vi "Outgoing Messages.vi"(8 "error in (no error)":errorcluster, 11 "Node Ptr":T3 format="%.0x") -> (0 "error out":errorcluster)   [LabVIEW 2009, in "NI-XNET Custom Device.lvlib"]
uses:
  NI-XNET Custom Device.lvlib
  <vilib>/NI VeriStand/Custom Device API/Custom Device Item Ref.ctl
  Add Selected.ctl
  Add All.ctl
  <vilib>/xnet/xnet.llb/XNET String To IO Name (Cluster).vi
  <vilib>/NI VeriStand/Custom Device API/Get Item Property (String).vi
  <vilib>/NI VeriStand/Custom Device API/Set Item Property (Variant).vi
  <vilib>/NI VeriStand/Custom Device API/Custom Device API.lvlib
  Program Files/National Instruments/LabVIEW 2009/resource/objmgr/xnet.rc
panel:
  out "Channel Assignment":u32(ring)=1 items=["A"=1, "B"=2, "A and B"=3]
  out "Cycle Repetition":u32
  out "Channel Assignments":u32[](array[numeric])
  out "Identifiers":u32[](array[numeric])
  out "In Cycle Repetitions?":bool
  out "Preamble":bool
  out "Startup":bool
  out "Sync":bool
  in  "Header 4":cluster{"Section Name 2":string}={"Section Name 2"="FlexRay Specific Settings"}
  in  "Frame Selection":i32(listbox)
  in  "Add All":T1
  in  "Header 3":cluster{"Section Name 2":string}={"Section Name 2"="Frame Timing"}
  in  "Header 2":cluster{"Section Name 2":string}={"Section Name 2"="Frame Settings"}
  out "Default Payload":u8[](array[numeric])
  out "Transmit Time":dbl
  out "Timing Type":u32(ring) items=["Cyclic Data", "Event Data", "Cyclic Remote", "Event Remote"]
  out "Extended Identifier?":bool
  out "Payload Length":u32
  out "Identifier":u32
  in  "Add Frame":T2
  in  "Header":cluster{"Section Name":string}={"Section Name"="Frame Selection"}
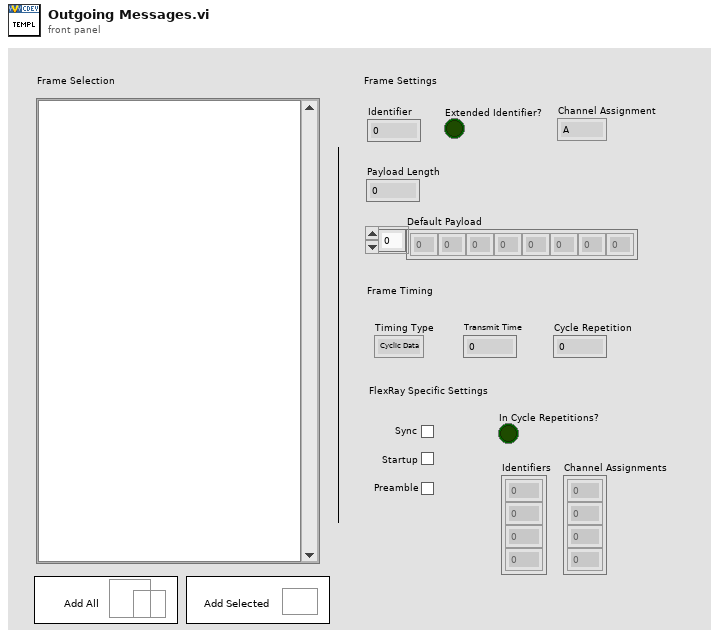
[diagram p1: front panel]
types:
  T1 = typedef "NI-XNET Custom Device.lvlib/Add All.ctl" = bool
  T2 = typedef "NI-XNET Custom Device.lvlib/Add Selected.ctl" = bool
  T3 = typedef "Custom Device API.lvlib/Custom Device Item Ref.ctl" = u64
  T4 = typedef "Custom Device API.lvlib/Custom Device Commands.ctl" = enum16{"Default", "Item renamed", "Shutdown"}
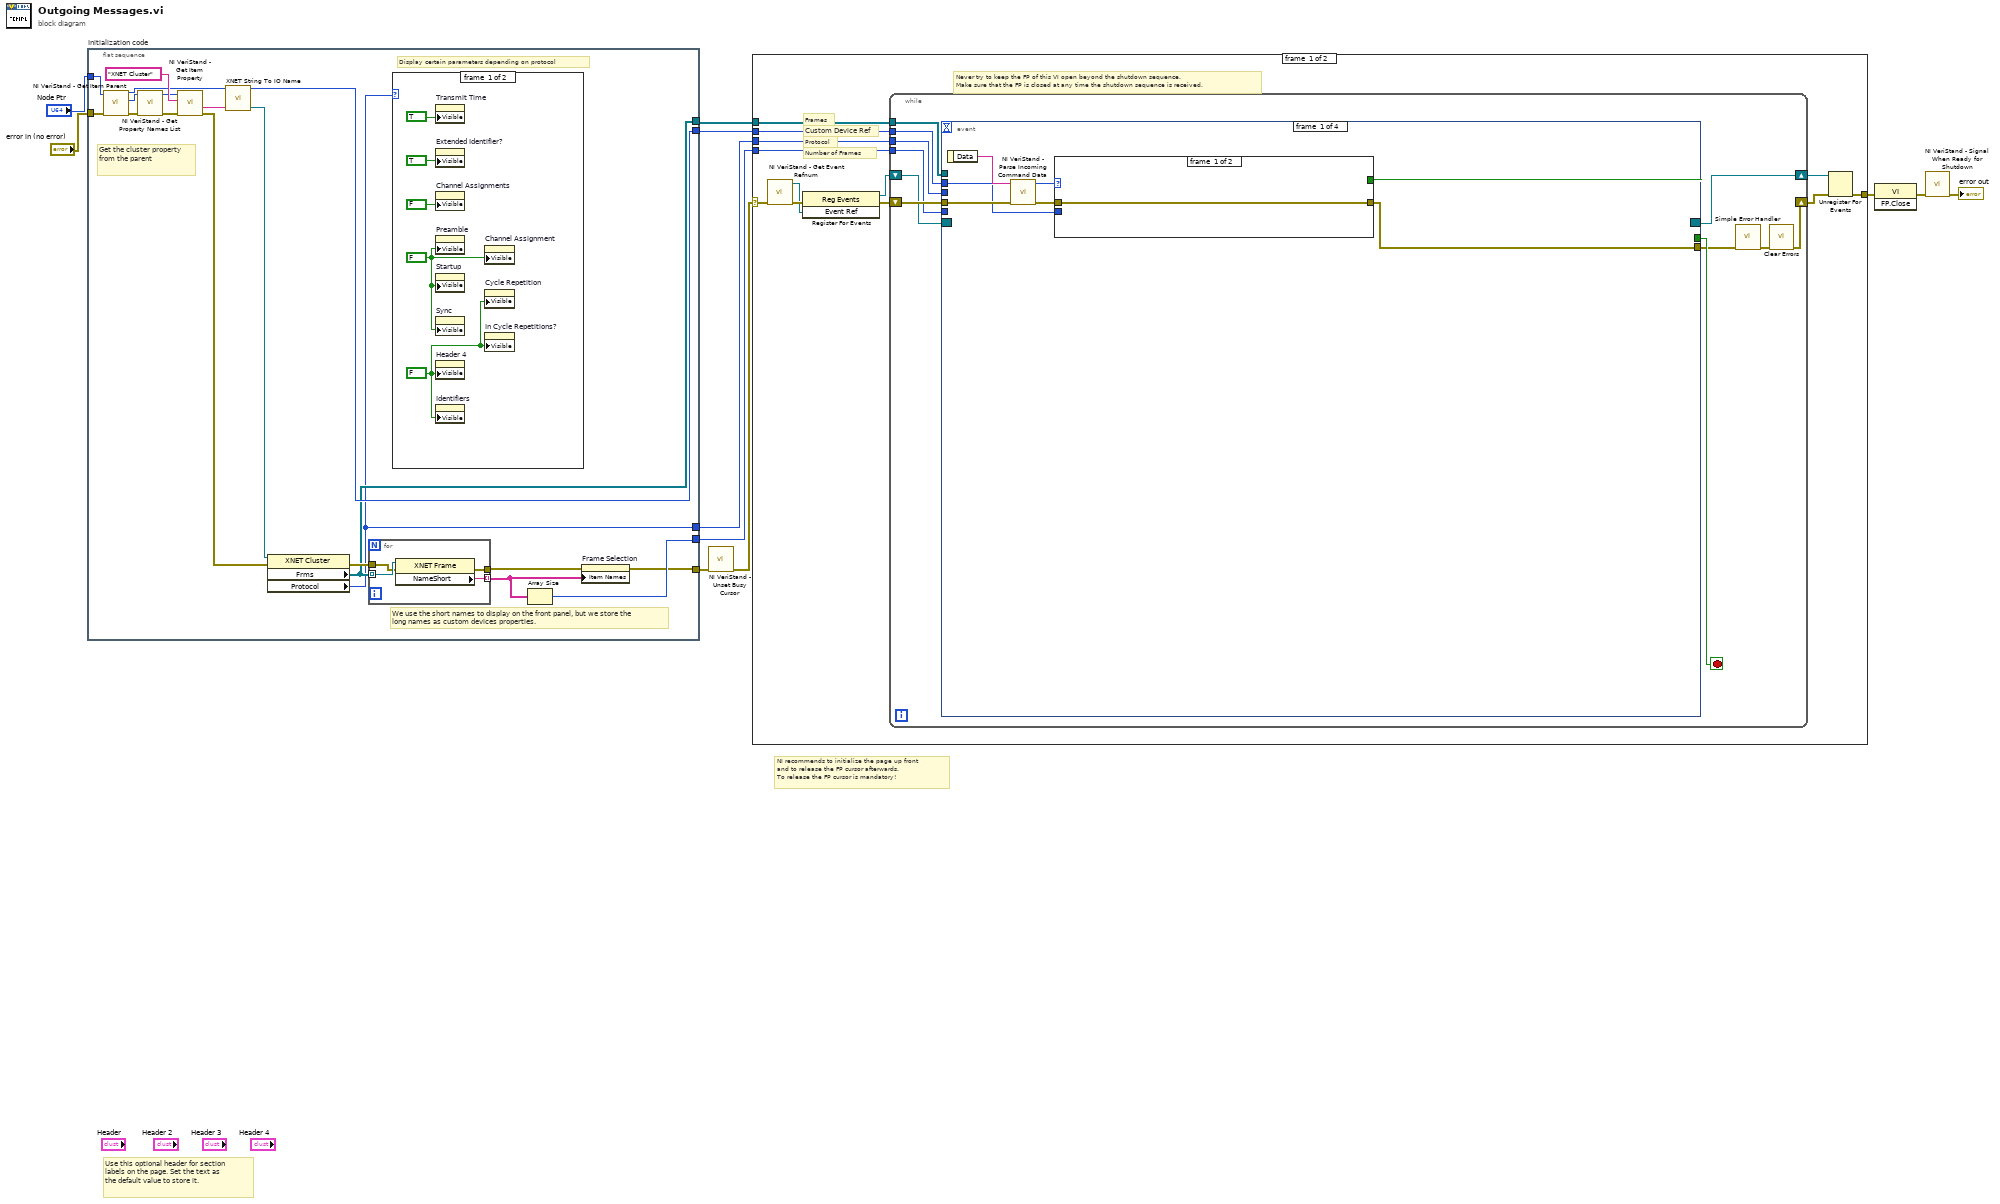
[diagram p0: block diagram]
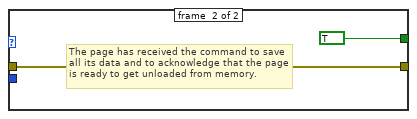
[diagram p2: hidden frame]
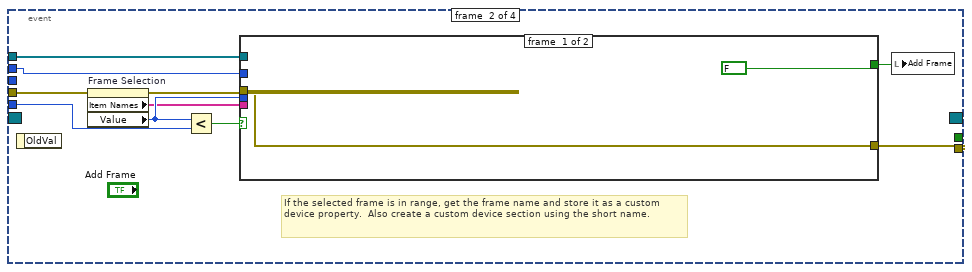
[diagram p3: hidden frame]
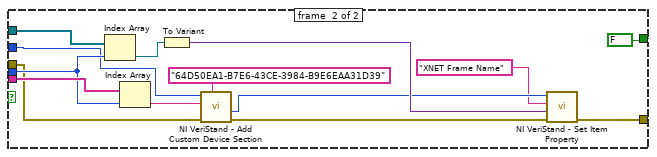
[diagram p4: hidden frame]
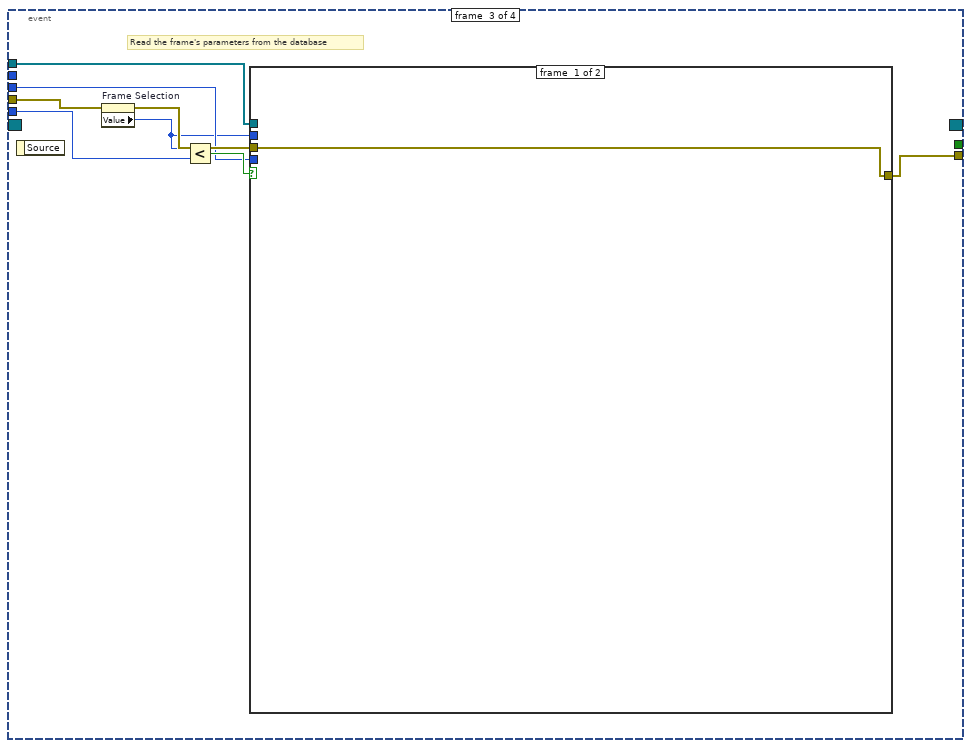
[diagram p5: hidden frame]
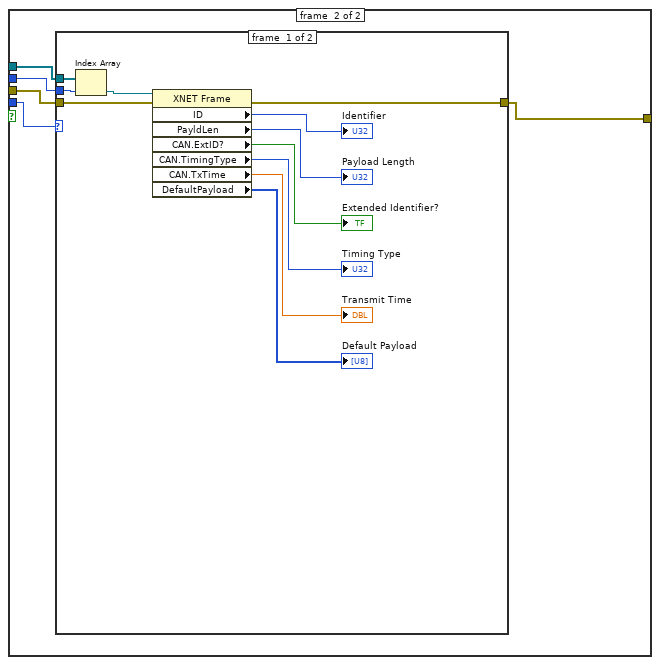
[diagram p6: hidden frame]
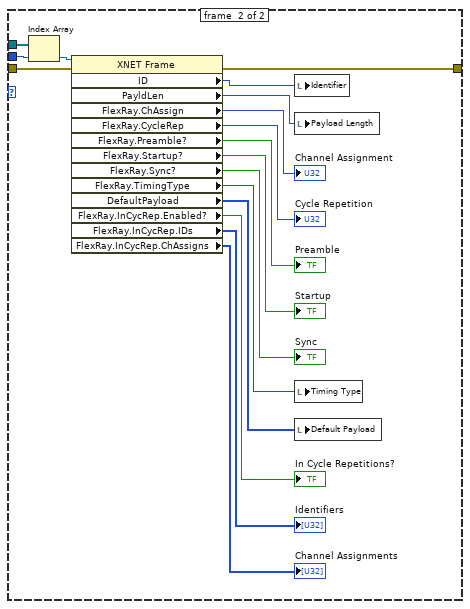
[diagram p7: hidden frame]
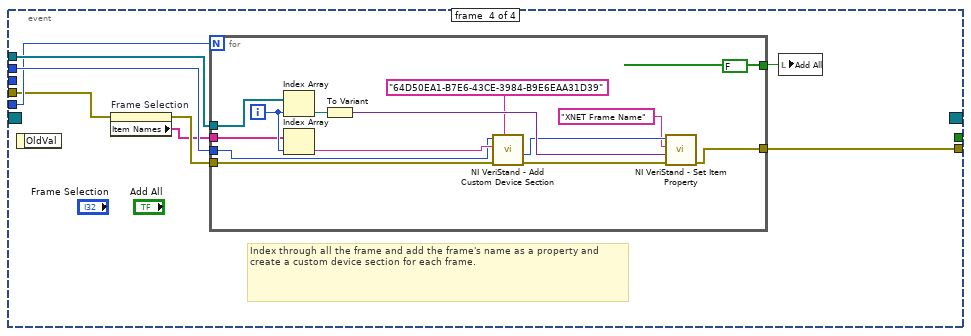
[diagram p8: hidden frame]
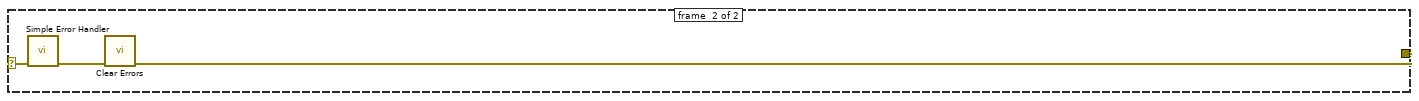
[diagram p9: hidden frame]
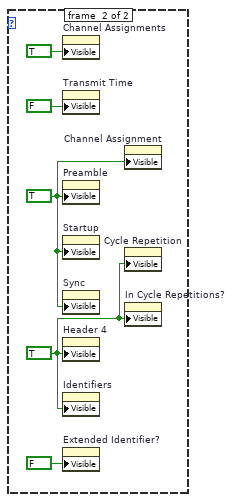
[diagram p10: hidden frame]
diagram:
  # "NI recommends to initialize the page up front\nand to release the FP cursor afterwards.\nTo release the FP cursor is mandatory!"
  # "Use this optional header for section labels on the page. Set the text as the default value to store it."
  n1 = flat-sequence "Initialization code" {
    tunnel: "error in (no error)" -> [w17]
    tunnel: "Node Ptr" -> [w16]
    tunnel: [w13] -> w7
    tunnel: [w21] -> w4
    tunnel: [w19] -> w3
    tunnel: [w18] -> w2
    tunnel: [w15] -> w1
    frame #0 {
      # "We use the short names to display on the front panel, but we store the \nlong names as custom devices properties."
      # "Display certain parameters depending on protocol"
      # "Get the cluster property from the parent"
      n2 = call <vilib>:"NI VeriStand - Get Item Parent.vi"("error in (no error)"=w17, "Parent Ref in"=w16) -> ("error out"=w27:errorcluster, "Parent Ref"=w28:T3, "Parent Ref out"=w21:T3)  [unwired: 6 in, 1 out]
      n3 = call <vilib>:"NI VeriStand - Get Property Names List.vi"("error in (no error)"=w27, "Item Ref in"=w28) -> ("error out"=w25:errorcluster, "Item Ref out"=w26:T3)  [unwired: 7 in, 1 out]
      n4 = call-poly <vilib>:"NI VeriStand - Get Item Property.vi"("error in (no error)"=w25, "Property Name"="XNET Cluster", "Item Ref in"=w26) -> ("error out"=w23:errorcluster, "Value"=w20:string)  [unwired: 5 in, 2 out]
      n5 = call-poly <vilib>:"XNET String To IO Name.vi"("string"=w20) -> ("XNET Cluster"=w24:refnum<k21>)  [unwired: 4 in]
      n6 = property class="XNET Cluster"(reference=w24, error in=w23) -> (error out=w22:errorcluster, "Frms"=w19:refnum<k21>[], "Protocol"=w15:u32)  [unwired: 1 out]
      n7 = for {
        tunnel: w19 -> [w43] mode=indexing
        tunnel: [w42] -> w14 mode=indexing
        tunnel: w22 -> [w41]
        tunnel: [w40] -> w12
        n8 = property class="XNET Frame"(reference=w43, error in=w41) -> (error out=w40:errorcluster, "NameShort"=w42:string)  [unwired: 1 out]
      }
      n9 = case shown="1" w15 {
        frame #0 {
          w33 = FALSE ("Visible")
          w34 = FALSE ("Visible")
          n10 = property on="Transmit Time" class="DigNum (strict)"("Visible"=TRUE) -> ()  [unwired: 2 in, 2 out]
          n11 = property on="Extended Identifier?" class="Bool (strict)"("Visible"=TRUE) -> ()  [unwired: 2 in, 2 out]
          n12 = property on="Channel Assignments" class="Arr (strict)"("Visible"=FALSE) -> ()  [unwired: 2 in, 2 out]
          n13 = property on="Preamble" class="Bool (strict)"("Visible"=w33) -> ()  [unwired: 2 in, 2 out]
          n14 = property on="Startup" class="Bool (strict)"("Visible"=w33) -> ()  [unwired: 2 in, 2 out]
          n15 = property on="Sync" class="Bool (strict)"("Visible"=w33) -> ()  [unwired: 2 in, 2 out]
          n16 = property on="Header 4" class="Clust (strict)"("Visible"=w34) -> ()  [unwired: 2 in, 2 out]
          n17 = property on="Identifiers" class="Arr (strict)"("Visible"=w34) -> ()  [unwired: 2 in, 2 out]
          n18 = property on="Channel Assignment" class="Ring (strict)"("Visible"=w33) -> ()  [unwired: 2 in, 2 out]
          n19 = property on="Cycle Repetition" class="DigNum (strict)"("Visible"=w34) -> ()  [unwired: 2 in, 2 out]
          n20 = property on="In Cycle Repetitions?" class="Bool (strict)"("Visible"=w34) -> ()  [unwired: 2 in, 2 out]
        }
        frame #1 {
          w36 = TRUE ("Visible")
          w37 = TRUE ("Visible")
          n21 = property on="Channel Assignments" class="Arr (strict)"("Visible"=TRUE) -> ()  [unwired: 2 in, 2 out]
          n22 = property on="Transmit Time" class="DigNum (strict)"("Visible"=FALSE) -> ()  [unwired: 2 in, 2 out]
          n23 = property on="Preamble" class="Bool (strict)"("Visible"=w36) -> ()  [unwired: 2 in, 2 out]
          n24 = property on="Startup" class="Bool (strict)"("Visible"=w36) -> ()  [unwired: 2 in, 2 out]
          n25 = property on="Sync" class="Bool (strict)"("Visible"=w36) -> ()  [unwired: 2 in, 2 out]
          n26 = property on="Header 4" class="Clust (strict)"("Visible"=w37) -> ()  [unwired: 2 in, 2 out]
          n27 = property on="Identifiers" class="Arr (strict)"("Visible"=w37) -> ()  [unwired: 2 in, 2 out]
          n28 = property on="Extended Identifier?" class="Bool (strict)"("Visible"=FALSE) -> ()  [unwired: 2 in, 2 out]
          n29 = property on="Channel Assignment" class="Ring (strict)"("Visible"=w36) -> ()  [unwired: 2 in, 2 out]
          n30 = property on="Cycle Repetition" class="DigNum (strict)"("Visible"=w37) -> ()  [unwired: 2 in, 2 out]
          n31 = property on="In Cycle Repetitions?" class="Bool (strict)"("Visible"=w37) -> ()  [unwired: 2 in, 2 out]
        }
      }
      n32 = Array Size(array=w14) -> (size(s)=w18:i32)
      n33 = property on="Frame Selection" class="LstBox (strict)"(error in=w12, "Item Names"=w14) -> (error out=w13:errorcluster)  [unwired: 1 in, 1 out]
    }
  }
  n34 = call <vilib>:"NI VeriStand - Unset Busy Cursor.vi"("error in (no error)"=w7) -> ("error out"=w6:errorcluster)  [unwired: 10 out]
  n35 = case shown="No Error" w6 {
    selector: w6 -> [w47 w169]
    tunnel: [w52 w167] -> w11
    tunnel: w4 -> [w48 _]
    tunnel: w3 -> [w46 _]
    tunnel: w2 -> [w45 _]
    tunnel: w1 -> [w44 _]
    frame #0 {
      # "Number of Frames"
      # "Custom Device Ref"
      # "Protocol"
      # "Frames"
      # "Never try to keep the FP of this VI open beyond the shutdown sequence.\nMake sure that the FP is closed at any time the shutdown sequence is received."
      n36 = call <vilib>:"NI VeriStand - Get Event Refnum.vi"("error in (no error)"=w47) -> ("error out"=w55:errorcluster, "Event Ref"=w51:refnum<user-event>)  [unwired: 9 out]
      n37 = register-events(error in=w55, w51) -> (reference out=w49:refnum<event-registration>, error out=w50:errorcluster)  [unwired: 1 in]
      n38 = while {
        tunnel: w48 -> [w60]
        shift-right: [w61] -> w53
        shift-left: w50 -> [w65]
        shift-right: [w66] -> w54
        shift-left: w49 -> [w64]
        tunnel: w46 -> [w59]
        tunnel: w45 -> [w58]
        tunnel: w44 -> [w56]
        stop <- w63 stop-if-true
        n39 = event shown="[2] \"Frame Selection\": Value Change;  \"Frame Selection\": Mouse Down;  \"Frame Selection\": Key Down;  \"Frame Selection\": Key Up" {
          selector: w64 -> [_ _ _ _]
          dyn-events: [_ _ _ _] -> w66
          timeout: _ -> [_ _ _ _]
          tunnel: w65 -> [w73 w81 w105 w148]
          tunnel: [w69 _ _ _] -> w63
          tunnel: [w67 w79 w106 w145] -> w57
          tunnel: w60 -> [w68 w86 _ w152]
          tunnel: w59 -> [_ w85 w110 w151]
          tunnel: w58 -> [_ w84 w109 w150]
          tunnel: w56 -> [_ _ w104 _]
          event #0 {
            n40 = event-data() -> ("Data"=w72:string)  [unwired: 1 out]
            n41 = call <vilib>:"NI VeriStand - Parse Incoming Command Data.vi"("error in (no error)"=w73, "Data"=w72) -> ("error out"=w71:errorcluster, "Action"=w70:T4)  [unwired: 8 out]
            n42 = case shown="\"Shutdown\"" w70 {
              tunnel: w71 -> [w74 w75]
              tunnel: [_ TRUE] -> w69
              tunnel: [w74 w75] -> w67
              tunnel: w68 -> [_ _]
              frame #0 {
              }
              frame #1 {
                # "The page has received the command to save all its data and to acknowledge that the page is ready to get unloaded from memory."
              }
            }
          }
          event #1 {
            # "If the selected frame is in range, get the frame name and store it as a custom device property.  Also create a custom device section using the short name."
            n43 = event-data() -> ()  [unwired: 2 out]
            n44 = property on="Frame Selection" class="LstBox (strict)"(error in=w81) -> (error out=w82:errorcluster, "Item Names"=w77:string[], "Value"=w78:i32)  [unwired: 1 in, 1 out]
            n45 = Less?(x=w78, y=w84) -> (x < y?=w83:bool)
            n46 = case shown="True" w83 {
              tunnel: w86 -> [_ w92]
              tunnel: w77 -> [_ w102]
              tunnel: w85 -> [_ w101]
              tunnel: w78 -> [_ w100]
              tunnel: w82 -> [w88 w91]
              tunnel: [w88 w89] -> w79
              tunnel: [FALSE ("Add Frame") FALSE ("Add Frame")] -> w80
              frame #0 {
              }
              frame #1 {
                n47 = Index Array(array=w101, index=w100) -> (element=w94:refnum<k21>)
                n48 = Index Array(array=w102, index=w100) -> (element=w93:string)
                n49 = To Variant(anything=w94) -> (Variant=w98:variant)
                n50 = call <vilib>:"NI VeriStand - Add Custom Device Section.vi"("GUID (Default Section)"="64D50EA1-B7E6-43CE-3984-B9E6EAA31D39", "error in (no error)"=w91, "Section Name"=w93, "Parent Ref in"=w92) -> ("error out"=w90:errorcluster, "Section Ptr"=w97:T3)  [unwired: 5 in, 1 out]
                n51 = call-poly <vilib>:"NI VeriStand - Set Item Property.vi"("error in (no error)"=w90, "Value"=w98, "Property Name"="XNET Frame Name", "Item Ref in"=w97) -> ("error out"=w89:errorcluster)  [unwired: 5 in, 2 out]
              }
            }
            n52 = local write "Add Frame"(w80) -> ()
          }
          event #2 {
            # "Read the frame's parameters from the database"
            n53 = event-data() -> ()  [unwired: 2 out]
            n54 = property on="Frame Selection" class="LstBox (strict)"(error in=w105) -> (error out=w107:errorcluster, "Value"=w103:i32)  [unwired: 1 in, 1 out]
            n55 = Less?(x=w103, y=w109) -> (x < y?=w108:bool)
            n56 = case shown="True" w108 {
              tunnel: w110 -> [_ w116]
              tunnel: w103 -> [_ w115]
              tunnel: w107 -> [w111 w114]
              tunnel: [w111 w113] -> w106
              tunnel: w104 -> [_ w112]
              frame #0 {
              }
              frame #1 {
                n57 = case shown="0, Default" w112 {
                  tunnel: w116 -> [w127 w144]
                  tunnel: w115 -> [w126 w143]
                  tunnel: w114 -> [w125 w141]
                  tunnel: [w124 w140] -> w113
                  frame #0 {
                    n58 = Index Array(array=w127, index=w126) -> (element=w123:refnum<k21>)
                    n59 = property class="XNET Frame"(reference=w123, error in=w125) -> (error out=w124:errorcluster, "ID"=→"Identifier":u32, "PayldLen"=→"Payload Length":u32, "CAN.ExtID?"=→"Extended Identifier?":bool, "CAN.TimingType"=→"Timing Type":u32, "CAN.TxTime"=→"Transmit Time":dbl, "DefaultPayload"=→"Default Payload":u8[])  [unwired: 1 out]
                  }
                  frame #1 {
                    n60 = Index Array(array=w144, index=w143) -> (element=w142:refnum<k21>)
                    n61 = property class="XNET Frame"(reference=w142, error in=w141) -> (error out=w140:errorcluster, "ID"=w139:u32, "PayldLen"=w138:u32, "FlexRay.ChAssign"=→"Channel Assignment":u32, "FlexRay.CycleRep"=→"Cycle Repetition":u32, "FlexRay.Preamble?"=→"Preamble":bool, "FlexRay.Startup?"=→"Startup":bool, "FlexRay.Sync?"=→"Sync":bool, "FlexRay.TimingType"=w130:u32, "DefaultPayload"=w129:u8[], "FlexRay.InCycRep.Enabled?"=→"In Cycle Repetitions?":bool, "FlexRay.InCycRep.IDs"=→"Identifiers":u32[], "FlexRay.InCycRep.ChAssigns"=→"Channel Assignments":u32[])  [unwired: 1 out]
                    n62 = local write "Identifier"(w139) -> ()
                    n63 = local write "Payload Length"(w138) -> ()
                    n64 = local write "Timing Type"(w130) -> ()
                    n65 = local write "Default Payload"(w129) -> ()
                  }
                }
              }
            }
          }
          event #3 {
            # "Index through all the frame and add the frame's name as a property and create a custom device section for each frame."
            n66 = event-data() -> ()  [unwired: 2 out]
            n67 = property on="Frame Selection" class="LstBox (strict)"(error in=w148) -> (error out=w147:errorcluster, "Item Names"=w146:string[])  [unwired: 1 in, 1 out]
            n68 = for {
              N: w150 -> [_]
              tunnel: w152 -> [w158]
              tunnel: w151 -> [w166]
              tunnel: w147 -> [w157]
              tunnel: [FALSE ("Add All")] -> w149
              tunnel: w146 -> [w154]
              tunnel: [w153] -> w145
              i -> [w165]
              n69 = Index Array(array=w166, index=w165) -> (element=w156:refnum<k21>)
              n70 = Index Array(array=w154, index=w165) -> (element=w159:string)
              n71 = To Variant(anything=w156) -> (Variant=w163:variant)
              n72 = call <vilib>:"NI VeriStand - Add Custom Device Section.vi"("GUID (Default Section)"="64D50EA1-B7E6-43CE-3984-B9E6EAA31D39", "error in (no error)"=w157, "Section Name"=w159, "Parent Ref in"=w158) -> ("error out"=w164:errorcluster, "Section Ptr"=w162:T3)  [unwired: 5 in, 1 out]
              n73 = call-poly <vilib>:"NI VeriStand - Set Item Property.vi"("error in (no error)"=w164, "Value"=w163, "Property Name"="XNET Frame Name", "Item Ref in"=w162) -> ("error out"=w153:errorcluster)  [unwired: 5 in, 2 out]
            }
            n74 = local write "Add All"(w149) -> ()
          }
        }
        n75 = call <vilib>:"Simple Error Handler.vi"("error in (no error)"=w57) -> ("error out"=w62:errorcluster)  [unwired: 1 in, 7 out]
        n76 = call <vilib>:"Clear Errors.vi"("error in (no error)"=w62) -> ("error out"=w61:errorcluster)  [unwired: 6 out]
      }
      n77 = Unregister For Events(event registration refnum=w54, error in=w53) -> (error out=w52:errorcluster)
    }
    frame #1 {
      n78 = call <vilib>:"Simple Error Handler.vi"("error in (no error)"=w169) -> ("error out"=w168:errorcluster)  [unwired: 1 in, 7 out]
      n79 = call <vilib>:"Clear Errors.vi"("error in (no error)"=w168) -> ("error out"=w167:errorcluster)  [unwired: 6 out]
    }
  }
  n80 = invoke class="VI" method="FP.Close"(error in=w11) -> (error out=w10:errorcluster)  [unwired: 2 in, 2 out]
  n81 = call <vilib>:"NI VeriStand - Signal When Ready for Shutdown.vi"("error in (no error)"=w10) -> ("error out"=→"error out":errorcluster)  [unwired: 10 out]
